vi "Team Index.vi"(11 "Square in":refnum<class "Square.lvclass">) -> (2 "Team Index":i32)   [LabVIEW 2020, in "SquareBattle.lvlib" / "Square.lvclass"]
uses:
  Square.lvclass
  Square.lvclass/Square.ctl
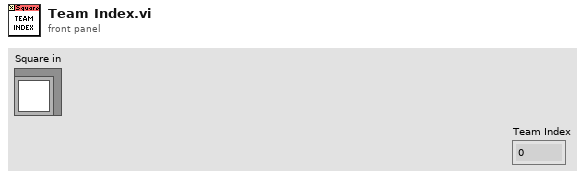
[diagram p1: front panel]
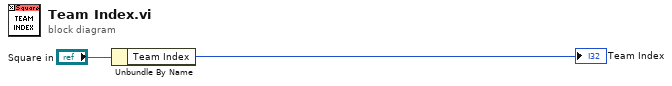
[diagram p0: block diagram]
diagram:
  n1 = Unbundle By Name("Square in") -> ("Team Index"=→"Team Index":i32)
